vi "shift visible array down four.vi"(8 "error in (no error)":errorcluster, 11 "Array in":refnum<vi>) -> (0 "error out":errorcluster, 3 "Array out":refnum<vi>)   [LabVIEW 2014, in "PID Module editor node.lvclass"]
doc: "This VI shifts the visible portion of the PID array down 4 elements"
uses:
  PID Module editor node.lvclass
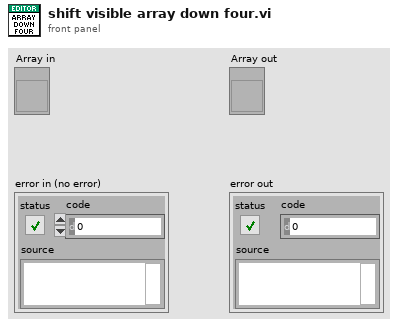
[diagram p1: front panel]
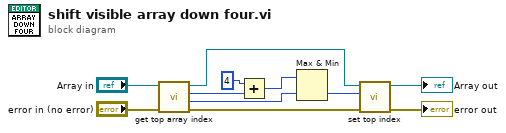
[diagram p0: block diagram]
diagram:
  n1 = call "get top array index.vi"("error in (no error)"="error in (no error)", "Array in"="Array in") -> ("error out"=w5:errorcluster, "last value index"=w1:u32, "top index"=w3:u32, "Array out"=w9:refnum<vi>)  [unwired: 6 in]
  n2 = Add(x=u32 4 ("y"), y=w3) -> (x+y=w2:u32)
  n3 = Max & Min(x=w2, y=w1) -> (min(x,y)=w10:u32)  [unwired: 1 out]
  n4 = call "set top index.vi"("error in (no error)"=w5, "Numeric"=w10, "Array in"=w9) -> ("error out"=→"error out":errorcluster, "Array out"=→"Array out":refnum<vi>)  [unwired: 7 in]
